vi "FPGA cRIOMain_v6.vi"() -> ()   [LabVIEW 2019]
doc: "Main FPGA VI\nUse the bitfile generated by this VI in the real-time code.\n\nv5: Use 16-pt MA filter in AI loop"
uses:
  TypeDefs/AO mode TabCtrl.ctl
  TypeDefs/SamplingModeEnum.ctl
  TypeDefs/AI_channelEnum.ctl
  <vilib>/Platform/TimedLoop/XDataNode/timing_clust.ctl
  <vilib>/Platform/TimedLoop/XDataNode/nitl_modes.ctl
  <vilib>/Platform/TimedLoop/XDataNode/wakeup.ctl
  <vilib>/rvi/Emulation/niFpgaGetClockAttributes.vi
  <vilib>/rvi/Emulation/niFpgaSctlEmulationGetInTimedLoop.vi
  <vilib>/rvi/Emulation/niFpgaEmulationReportErrorSimple.vi
  <vilib>/rvi/eio/common/nirviEmuTemplateMethod_errors.vi
  <vilib>/rvi/Emulation/niFpgaEmulationIsFPGAContextNoSignature.vi
  <vilib>/rvi/DataTransferAndStorage/Container/Common/niFpgaContainerGetUniqueNameForEmu.vi
  <vilib>/rvi/Memory/Memory_Emulation/niFpgaMemoryEmulationCacheClearOnFirstRun.vi
  <vilib>/rvi/Memory/Memory_Emulation/nirvimemoryEmulationManagerCache_MakeExclusive.vi
  <vilib>/rvi/Memory/Memory_Emulation/niFpgaMemoryEmulationValidateCache.vi
  <vilib>/rvi/Memory/Memory_Emulation/nirvimemoryEmulationManagerCache_InsertValue.vi
  <vilib>/Utility/error.llb/Clear Errors.vi
  <vilib>/rvi/Memory/Memory_Emulation/nirvimemoryEmulationManagerCache_ReleaseExclusive.vi
  <vilib>/rvi/Memory/Memory_Emulation/nirvimemoryEmulationManagerCache_GetValue.vi
  <vilib>/rvi/Memory/Memory_Emulation/nirvimemoryEmulationManagerCache_SetValue.vi
  <vilib>/rvi/Emulation/niFpgaProcessEmulError.vi
  <vilib>/rvi/errors/niFpgaSetErrorForExecOnDevCompSimple.vi
  <vilib>/rvi/eio/common/nirviEmuReportErrorAndStop.vi
  <vilib>/rvi/FIFO/Fifo_Resource/nirvififoEmulationSetSize.vi
  <vilib>/rvi/FIFO/Fifo_Resource/nirviFifoEmulationQueueMgr.vi
  <instcachedir>/0/nirviFifoEmulationQueueMgr_E5CAEC123FF24DC58D834DCA3CDAA9B5.lvgen/nirviFifoEmulationQueueMgr_E5CAEC123FF24DC58D834DCA3CDAA9B5_000.vi
  <vilib>/rvi/FIFO/Fifo_Resource/nirvififoEmulationDetermineInputValidOut.vi
  <vilib>/rvi/FIFO/Fifo_Resource/nirvififoEmulationCreateLock.vi
  <vilib>/rvi/FIFO/Fifo_Resource/nirvififoEmulationObtainLock.vi
  <vilib>/rvi/FIFO/Fifo_Resource/nirvififoEmulationReleaseLock.vi
  <vilib>/rvi/occurrence/nirviWaitOnOccurrenceBase.vi
  <vilib>/rvi/errors/nirviReportUnexpectedCaseInternalError.vi
  <vilib>/rvi/errors/nirviReportUnexpectedCaseInternalError (U32).vi
  <vilib>/rvi/Emulation/niFpgaCriticalErrorInLSC.vi
  <instcachedir>/0/nirviFifoEmulationQueueMgr_E5CAEC123FF24DC58D834DCA3CDAA9B5.lvgen/nirviFifoEmulationQueueMgr_E5CAEC123FF24DC58D834DCA3CDAA9B5_006.vi
  <vilib>/rvi/Analysis/common/codeGenErrors/XNode/niFpgaXNodeCodeGenErrorHandle.vi
  <vilib>/eio/EIONode/EIONode.xnode
  <vilib>/rvi/DataTransferAndStorage/Container/XNode/niFpgaContainer.xnode
  <vilib>/rvi/DataTransferAndStorage/Register/Emulation/niFpgaRegisterEmulation.vi
  <vilib>/rvi/FIFO/Fifo_Resource/nirvififoEmulationWrite.vi
  <vilib>/rvi/FIFO/Fifo_Resource/nirvififoEmulationRead.vi
  <vilib>/rvi/Analysis/measure/butterworth/XNode/niFpgaButterworthFilter.xnode
  <vilib>/rvi/FXPMathLib/FxpMul/XNode/nifxpmath_Multiplier.xnode
  <vilib>/rvi/Analysis/measure/LMRsmpl/XNode/niFPGA Rational Resampler.xnode
  <vilib>/Platform/TimedLoop/XDataNode/XDataNode.xnode
  FPGA functions/FPGA functions.lvlib
  <vilib>/rvi/FXPMathLib/sim/FxpSim.dll
  <vilib>/Platform/TimedLoop/XDataNode/XDNodeRunTimeDep.lvlib
panel:
  out "AI M loop time [ticks]":u32
  out "FPGA AI DMA\nOverflow?":bool
  out "AI Processing\nLoop Rate to high?":bool
  in  "AI Process Time [ticks]":u32=121
  in  "Select Channel":T1
  out "Unable to\nsample at desired\nSample Rate?":bool
  out "Processing Loop time [ticks]":u32
  in  "Scaled Butterworth Coeffs_AI_Proc":i32[](array[numeric])=[-1036986264, 2110353124, 93741, -1058362983, 2131726043, 94691]
  in  "Sampling Mode":T2
  in  "AO mode":T3
  in  "AO Out [V]":fxp<+/-,18,5> format="%#.6g"
  in  "AO enable?":bool
  out "AI In [V]":fxp<+/-,26,5> format="%#.6g"
  out "FPGA AO DMA\nOverflow?":bool
  out "Int. Output":fxp<+/-,20,5> format="%.17g"
  out "Raw AI Input":fxp<+/-,26,5> format="%.21g"
  in  "Sample Time [ticks]":u32=121
  out "AO Loop time [ticks]":u32
  out "AI Loop time [ticks]":u32
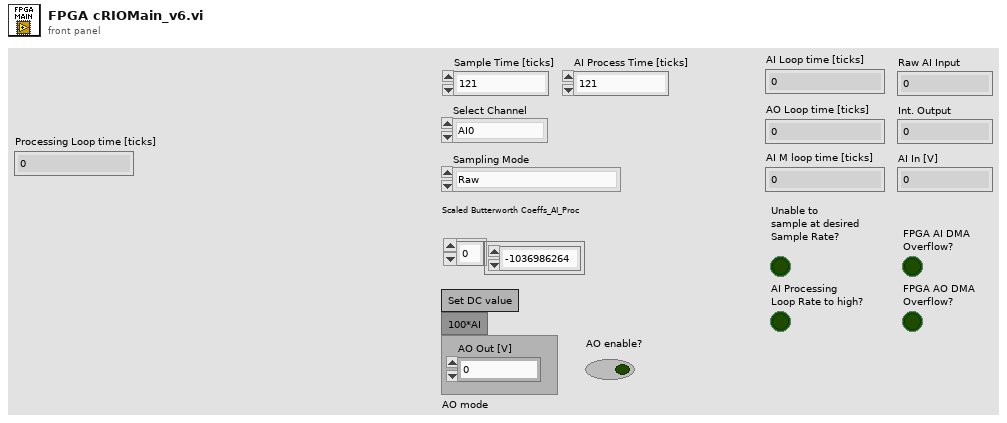
[diagram p1: front panel]
types:
  T1 = typedef "AI_channelEnum.ctl" = enum16{"AI0", "AI1", "AI2", "AI3"}
  T2 = typedef "SamplingModeEnum.ctl" = enum16{"Raw", "4pt MA (AI)", "LPF (Proc.)", "4pt MA (AI) + LPF (Proc.)", "4pt MA (Proc.) + LPF (Proc.)"}
  T3 = typedef "AO mode TabCtrl.ctl" = enum32{"Set DC value", "100*AI"}
  T4 = typedef "XDNodeRunTimeDep.lvlib/timing_clust.ctl" = cluster{"Expected End [f-1]":u64, "Actual End [f-1]":u64, "Finished Late? [f-1]":bool, "Expected End [i-1]":u64, "Actual End [i-1]":u64, "Finished Late? [i-1]":bool, "Expected Start [i]":u64, "Actual Start [i]":u64, "Expected Start [f]":u64, "Actual Start [f]":u64, "Source Name":string, "Structure Name":string, "Period":i64, "Deadline":i64, "Offset":i64, "Start":i64, "Priority":i32, "Timeout":i32, "Mode":T5, "Wakeup Reason":T6, "Error":errorcluster, "Source Type":string, "Secondary Source Type":string, "Global End Time":u64, "Global Start Time":u64, "Frame Duration":u64, "Iteration Duration":u64, "Assigned CPU":i32, "I/O Scan Engine Mode":u32}
  T5 = typedef "XDNodeRunTimeDep.lvlib/nitl_modes.ctl" = enum32{"No Change", "Process missed periods, maintain original phase", "Discard missed periods, maintain original phase", "Process missed periods, ignore original phase", "Discard missed periods, ignore original phase"}
  T6 = typedef "XDNodeRunTimeDep.lvlib/wakeup.ctl" = enum32{"Normal", "Aborted", "Asynchronous wakeup", "Timing source error", "Timed loop error", "Timeout"}
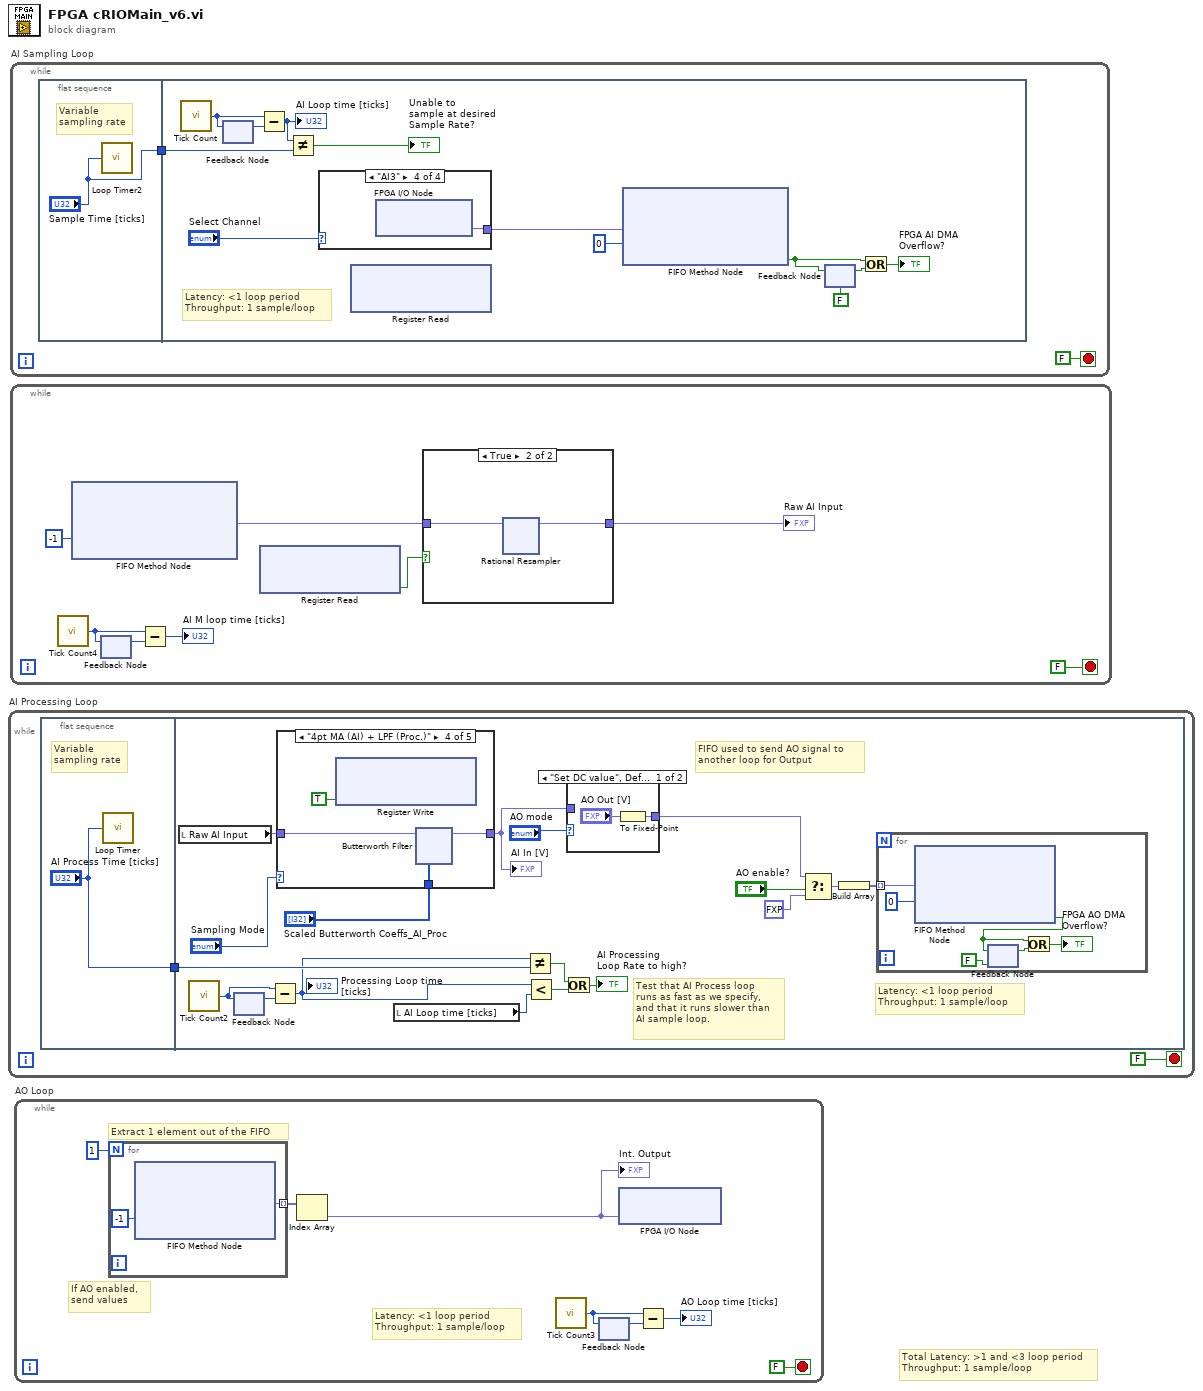
[diagram p0: block diagram]
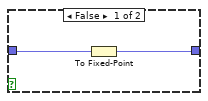
[diagram p2: hidden frame]
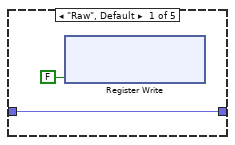
[diagram p3: hidden frame]
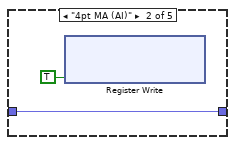
[diagram p4: hidden frame]
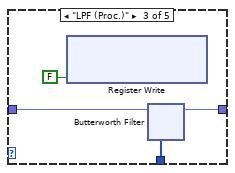
[diagram p5: hidden frame]
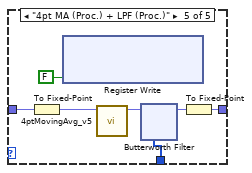
[diagram p6: hidden frame]
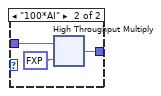
[diagram p7: hidden frame]
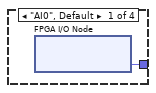
[diagram p8: hidden frame]
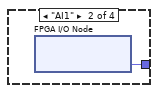
[diagram p9: hidden frame]
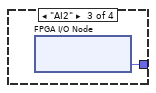
[diagram p10: hidden frame]
diagram:
  # "Total Latency: >1 and <3 loop period\nThroughput: 1 sample/loop"
  n1 = while "AI Processing Loop" {
    stop <- FALSE stop-if-true
    n2 = flat-sequence {
      tunnel: ["AI Process Time [ticks]"] -> w1
      tunnel: w1 -> [w5]
      frame #0 {
        # "Variable\nsampling rate"
        n3 = call "Loop Timer"("Count(Ticks)"="AI Process Time [ticks]") -> ()  [unwired: 1 out]
      }
      frame #1 {
        # "Test that AI Process loop\nruns as fast as we specify,\nand that it runs slower than \nAI sample loop."
        # "Latency: <1 loop period\nThroughput: 1 sample/loop"
        # "FIFO used to send AO signal to \nanother loop for Output"
        n4 = local read "Raw AI Input"() -> (w9:fxp<+/-,26,5>)
        n5 = call "Tick Count2"() -> ("Tick Count(Ticks)"=w20:u32)
        n6 = feedback #1() -> (w21:u32)  [unwired: 1 in]
        n7 = feedback-in #1(w20) -> ()
        n8 = Subtract(x=w20, y=w21) -> (x-y=w4:u32)
        "Processing Loop time [ticks]" <- w4
        n9 = case shown="\"4pt MA (AI) + LPF (Proc.)\"" "Sampling Mode" {
          tunnel: "Scaled Butterworth Coeffs_AI_Proc" -> [_ _ w29 w41 w56]
          tunnel: [w22 w24 w28 w40 w50] -> w18
          tunnel: w9 -> [w22 w24 w26 w38 w53]
          frame "Raw", Default {
            n10 = xnode ("Register Write")("Data"=FALSE) -> ()  [unwired: 1 in, 1 out]
          }
          frame "4pt MA (AI)" {
            n11 = xnode ("Register Write")("Data"=TRUE) -> ()  [unwired: 1 in, 1 out]
          }
          frame "LPF (Proc.)" {
            n12 = xnode ("Register Write")("Data"=FALSE) -> ()  [unwired: 1 in, 1 out]
            n13 = xnode "Butterworth Filter"("input data"=w26, "scaled coefficients"=w29) -> ("output data"=w28:fxp<+/-,26,5>)  [unwired: 1 in]
          }
          frame "4pt MA (AI) + LPF (Proc.)" {
            n14 = xnode ("Register Write")("Data"=TRUE) -> ()  [unwired: 1 in, 1 out]
            n15 = xnode "Butterworth Filter"("input data"=w38, "scaled coefficients"=w41) -> ("output data"=w40:fxp<+/-,26,5>)  [unwired: 1 in]
          }
          frame "4pt MA (Proc.) + LPF (Proc.)" {
            n16 = To Fixed-Point(number=w53) -> (fixed-point=w54:fxp<+/-,24,5>)  [unwired: 1 in]
            n17 = xnode ("Register Write")("Data"=FALSE) -> ()  [unwired: 1 in, 1 out]
            n18 = call "4ptMovingAvg_v5.vi"("Raw input"=w54) -> ("Avg. output"=w55:fxp<+/-,25,5>)  [unwired: 10 in]
            n19 = xnode "Butterworth Filter"("input data"=w55, "scaled coefficients"=w56) -> ("output data"=w51:fxp<+/-,25,5>)  [unwired: 1 in]
            n20 = To Fixed-Point(number=w51) -> (fixed-point=w50:fxp<+/-,26,5>)  [unwired: 1 in]
          }
        }
        "AI In [V]" <- w18
        n21 = local read "AI Loop time [ticks]"() -> (w10:u32)
        n22 = Not Equal?(x=w4, y=w5) -> (x != y?=w7:bool)
        n23 = Less?(x=w4, y=w10) -> (x < y?=w6:bool)
        n24 = Or(x=w7, y=w6) -> (x .or. y?=→"AI Processing\nLoop Rate to high?":bool)
        n25 = case shown="\"Set DC value\", Default" "AO mode" {
          tunnel: [w66 w67] -> w14
          tunnel: w18 -> [_ w69]
          frame "Set DC value", Default {
            n26 = To Fixed-Point(number="AO Out [V]") -> (fixed-point=w66:fxp<+/-,20,5>)  [unwired: 1 in]
          }
          frame "100*AI" {
            n27 = xnode ("High Throughput Multiply")("x"=w69, "y"=fxp<+,5,7> 100.0) -> ("x*y"=w67:fxp<+/-,20,5>)
          }
        }
        n28 = Select(t=w14, s="AO enable?", f=fxp<+/-,20,5> 0.0) -> (s? t:f=w19:fxp<+/-,20,5>)
        n29 = Build Array(w19) -> (w13:fxp<+/-,20,5>[])
        n30 = for {
          tunnel: w13 -> [w70] mode=indexing
          n31 = xnode ("FIFO Method Node")("Element"=w70, "Timeout"=0) -> ("Timed Out?"=w71:bool)  [unwired: 1 in, 1 out]
          n32 = feedback-in #2(w71) -> ()
          n33 = feedback #2(FALSE ("Timed Out?")) -> (w74:bool)
          n34 = Or(x=w71, y=w74) -> (x .or. y?=→"FPGA AO DMA\nOverflow?":bool)
        }
      }
    }
  }
  n35 = while "AI Sampling Loop" {
    stop <- FALSE stop-if-true
    n36 = flat-sequence {
      tunnel: ["Sample Time [ticks]"] -> w76
      tunnel: w76 -> [w87]
      frame #0 {
        # "Variable\nsampling rate"
        n37 = call "Loop Timer2"("Count(Ticks)"="Sample Time [ticks]") -> ()  [unwired: 1 out]
      }
      frame #1 {
        # "Latency: <1 loop period\nThroughput: 1 sample/loop"
        n38 = call "Tick Count"() -> ("Tick Count(Ticks)"=w90:u32)
        n39 = feedback #3() -> (w89:u32)  [unwired: 1 in]
        n40 = feedback-in #3(w90) -> ()
        n41 = Subtract(x=w90, y=w89) -> (x-y=w88:u32)
        "AI Loop time [ticks]" <- w88
        n42 = Not Equal?(x=w88, y=w87) -> (x != y?=→"Unable to\nsample at desired\nSample Rate?":bool)
        n43 = case shown="\"AI3\"" "Select Channel" {
          tunnel: [w91 w92 w93 w94] -> w84
          frame "AI0", Default {
            n44 = xnode "FPGA I/O Node"() -> ("Mod4/AI0"=w91:fxp<+/-,24,5>)  [unwired: 1 in, 1 out]
          }
          frame "AI1" {
            n45 = xnode "FPGA I/O Node"() -> ("Mod4/AI1"=w92:fxp<+/-,24,5>)  [unwired: 1 in, 1 out]
          }
          frame "AI2" {
            n46 = xnode "FPGA I/O Node"() -> ("Mod4/AI2"=w93:fxp<+/-,24,5>)  [unwired: 1 in, 1 out]
          }
          frame "AI3" {
            n47 = xnode "FPGA I/O Node"() -> ("Mod4/AI3"=w94:fxp<+/-,24,5>)  [unwired: 1 in, 1 out]
          }
        }
        n48 = xnode ("Register Read")() -> ()  [unwired: 1 in, 2 out]
        n49 = xnode ("FIFO Method Node")("Element"=w84, "Timeout"=0) -> ("Timed Out?"=w81:bool)  [unwired: 1 in, 1 out]
        n50 = feedback #4(FALSE ("Timed Out?")) -> (w83:bool)
        n51 = feedback-in #4(w81) -> ()
        n52 = Or(x=w81, y=w83) -> (x .or. y?=→"FPGA AI DMA\nOverflow?":bool)
      }
    }
  }
  n53 = while {
    stop <- FALSE stop-if-true
    n54 = call "Tick Count4"() -> ("Tick Count(Ticks)"=w98:u32)
    n55 = xnode ("FIFO Method Node")("Timeout"=-1) -> ("Element"=w100:fxp<+/-,24,5>)  [unwired: 1 in, 2 out]
    n56 = feedback #5() -> (w97:u32)  [unwired: 1 in]
    n57 = feedback-in #5(w98) -> ()
    n58 = Subtract(x=w98, y=w97) -> (x-y=→"AI M loop time [ticks]":u32)
    n59 = xnode ("Register Read")() -> ("Data"=w95:bool)  [unwired: 1 in, 1 out]
    n60 = case shown="True" w95 {
      tunnel: w100 -> [w103 w106]
      tunnel: [w104 w105] -> w99
      frame False {
        n61 = To Fixed-Point(number=w103) -> (fixed-point=w104:fxp<+/-,26,5>)  [unwired: 1 in]
      }
      frame True {
        n62 = xnode "Rational Resampler"("input data"=w106) -> ("output data"=w105:fxp<+/-,26,5>)  [unwired: 2 out]
      }
    }
    "Raw AI Input" <- w99
  }
  n63 = while "AO Loop" {
    stop <- FALSE stop-if-true
    # "Latency: <1 loop period\nThroughput: 1 sample/loop"
    # "If AO enabled, \nsend values"
    # "Extract 1 element out of the FIFO"
    n64 = for {
      N: 1 -> [_]
      tunnel: [w149] -> w143 mode=indexing
      n65 = xnode ("FIFO Method Node")("Timeout"=-1) -> ("Element"=w149:fxp<+/-,20,5>)  [unwired: 1 in, 2 out]
    }
    n66 = Index Array(array=w143) -> (element=w141:fxp<+/-,20,5>)  [unwired: 1 in]
    "Int. Output" <- w141
    n67 = call "Tick Count3"() -> ("Tick Count(Ticks)"=w146:u32)
    n68 = feedback #6() -> (w145:u32)  [unwired: 1 in]
    n69 = feedback-in #6(w146) -> ()
    n70 = xnode "FPGA I/O Node"("Mod3/AO1"=w141) -> ()  [unwired: 1 in, 1 out]
    n71 = Subtract(x=w146, y=w145) -> (x-y=→"AO Loop time [ticks]":u32)
  }
